vi "Python Object Reference to Pointer Sized Ref.vi"(1 "Refnum in":T1) -> (0 "Py Object":u64)   [LabVIEW 2020, in "G-Embedded-Python-Interpreter-Toolkit.lvlib"]
uses:
  G-Embedded-Python-Interpreter-Toolkit.lvlib
  Python Object Reference.ctl
  Python Object Type.ctl
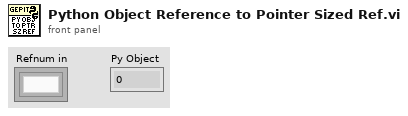
[diagram p1: front panel]
types:
  T1 = typedef "G-Embedded-Python-Interpreter-Toolkit.lvlib/Python Object Reference.ctl" = refnum<k1>
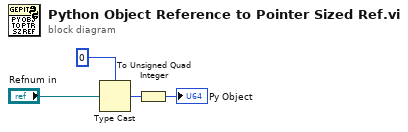
[diagram p0: block diagram]
diagram:
  n1 = Type Cast(type=u32 0, x="Refnum in") -> (*(type *) &x=w3:u32)
  n2 = To Unsigned Quad Integer(1:w3) -> (0:→"Py Object":u64)
